vi "Efficiency Calculation.vi"(8 "Current":dbl format="%#_13g", 9 "Voltage":dbl format="%#_13g", 10 "Flow":dbl format="%#_13g", 11 "Pressure":dbl format="%#_13g") -> (3 "%Efficiency":dbl)   [LabVIEW 2013]
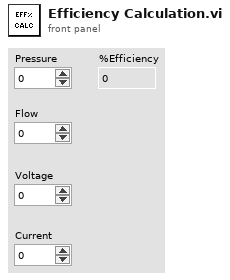
[diagram p1: front panel]
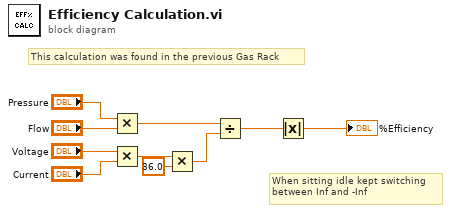
[diagram p0: block diagram]
diagram:
  # "When sitting idle kept switching\nbetween Inf and -Inf"
  # "This calculation was found in the previous Gas Rack"
  n1 = Multiply(x="Pressure", y="Flow") -> (x*y=w3:dbl)
  n2 = Multiply(x="Voltage", y="Current") -> (x*y=w6:dbl)
  n3 = Multiply(x=w6, y=36.0) -> (x*y=w4:dbl)
  n4 = Divide(x=w3, y=w4) -> (x/y=w2:dbl)
  n5 = Absolute Value(x=w2) -> (abs(x)=→"%Efficiency":dbl)
